vi "Test Throw error on space JSON input.vi"(11 "Test Case In":refnum<class "Test Strict Find Items as LV Type.lvclass">) -> (0 "error out":errorcluster, 3 "Test Case Out":refnum<class "Test Strict Find Items as LV Type.lvclass">)   [LabVIEW 2024, in "Test Strict Find Items as LV Type.lvclass"]
uses:
  Test Strict Find Items as LV Type.lvclass
  Test Strict Find Items as LV Type.lvclass/Test Strict Find Items as LV Type.ctl
  <vilib>/Astemes/LUnit/Test Case.lvclass
  e024d05f-1469-41e1-8c16-ce5a8bcc6b45.vi
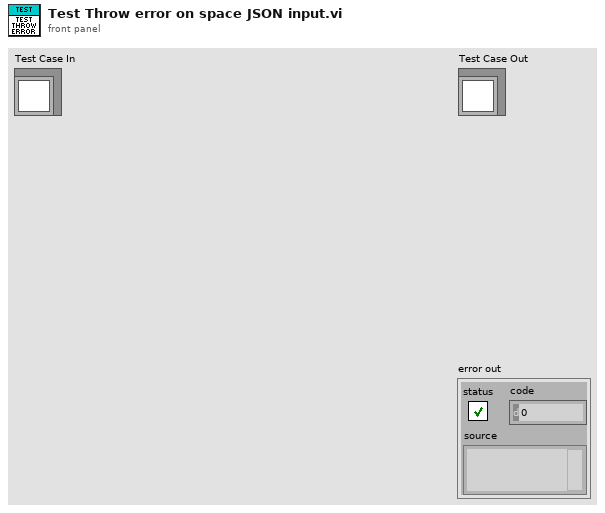
[diagram p1: front panel]
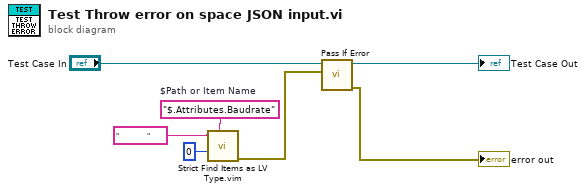
[diagram p0: block diagram]
diagram:
  w3 = "$.Attributes.Baudrate"  # $Path or Item Name
  n1 = call "Strict Find Items as LV Type.vim"("$Path or Item Name"=w3, "Data Type and Default Value"=u16 0, "<JSON>"="              ") -> ("error out"=w2:errorcluster)  [unwired: 6 in, 2 out]
  n2 = call <vilib>:"Pass If Error.vi"("Assert error"=w2, "LUnit Test Case In"="Test Case In") -> ("error out"=→"error out":errorcluster, "LUnit Test Case Out"=→"Test Case Out":refnum<class "Test Strict Find Items as LV Type.lvclass">)  [unwired: 8 in]
